vi "Do That Thang Core.vi"(7 "Test Executive Ref":refnum<data-value>, 8 "error in (no error)":errorcluster, 9 "Attributes Ref":refnum<data-value>, 11 "Iterate in":refnum<class "Iterate.lvclass">) -> (0 "error out":errorcluster)   [LabVIEW 2019, in "Nested Conditional in While Loop Example.lvlib" / "Iterate.lvclass"]
uses:
  <vilib>/gpm_packages/@cs/test-executive/Source/Sandbox/Nested Conditional in While Loop Example/Iterate/Iterate.lvclass
  <vilib>/gpm_packages/@cs/test-executive/Source/Test Executive/ITestExecutive/ITest Executive.lvclass
  <vilib>/gpm_packages/@cs/lookup-table/Source/LookupTable/LookupTable.lvclass
  <vilib>/gpm_packages/@cs/lookup-table/Source/LookupTable/LookupTable.lvclass/LookupTable.ctl
  f6d01b24-9f96-46a8-9a52-477756870b25.vi
  43d2138b-deef-4c25-90bd-110e8042b925.vi
  f45db74b-0238-44c3-965f-22bb3648defb.vi
  <vilib>/gpm_packages/@cs/lookup-table/Source/LookupTable/Read Table Reference.vi
  f6d01b24-9f96-46a8-9a52-477756870b25.vi/a19a1958-3e3f-4e6a-964b-fde1466acadd.vi
  <vilib>/Utility/error.llb/Error Cluster From Error Code.vi
  <vilib>/gpm_packages/@cs/test-executive/Source/Test Executive/TestExecutive Ref/TestExecutive Ref.lvclass
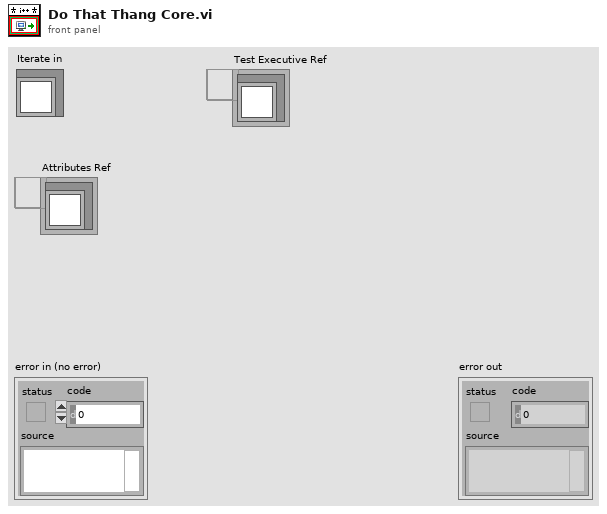
[diagram p1: front panel]
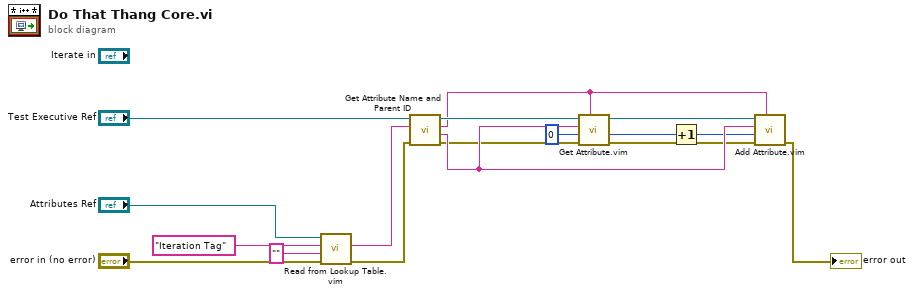
[diagram p0: block diagram]
diagram:
  n1 = call "Read from Lookup Table.vim"("error in (no error)"="error in (no error)", "Type"="", "Item Name"="Iteration Tag", "LookupTable Reference"="Attributes Ref") -> ("error out"=w4:errorcluster, "Value"=w8:string)  [unwired: 4 in, 2 out]
  n2 = call <vilib>:"Get Attribute Name and Parent ID.vi"("error in (no error)"=w4, "Tag"=w8, "Test Executive Ref"="Test Executive Ref") -> ("error out"=w3:errorcluster, "Attribute Name"=w11:string, "Parent ID"=w12:string, "Test Executive Ref out"=w15:refnum<data-value>)  [unwired: 5 in]
  n3 = call "Get Attribute.vim"("ID"=w12, "error in (no error)"=w3, "Type"=0, "Attribute Name"=w11, "Test Executive Ref"=w15) -> ("error out"=w2:errorcluster, "Attribute"=w10:i32, "Test Executive Ref out"=w13:refnum<data-value>)  [unwired: 2 in, 2 out]
  n4 = Increment(x=w10) -> (x+1=w9:i32)
  n5 = call "Add Attribute.vim"("ID"=w12, "error in (no error)"=w2, "Attribute"=w9, "Attribute Name"=w11, "Test Executive Ref"=w13) -> ("error out"=→"error out":errorcluster)  [unwired: 3 in, 3 out]
